vi "Initialise all lasers.vi"() -> (4 "455 laser":refnum<visa-resource-name>, 6 "488 laser":refnum<visa-resource-name>, 8 "561 laser":refnum<visa-resource-name>, 10 "647 laser":refnum<visa-resource-name>, 15 "error out":errorcluster)   [LabVIEW 2017]
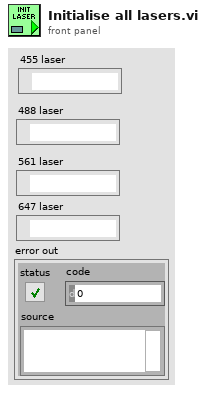
[diagram p1: front panel]
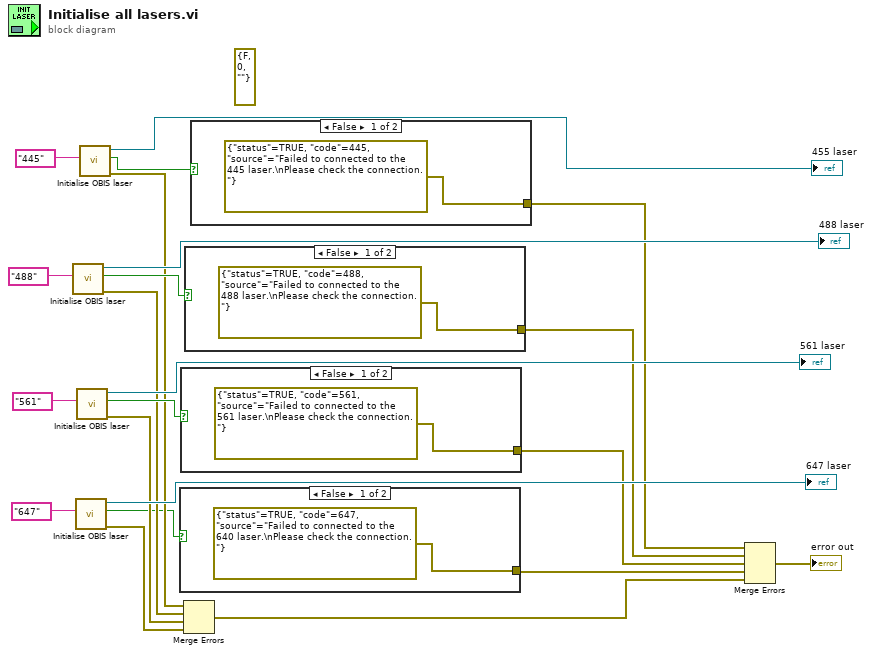
[diagram p0: block diagram]
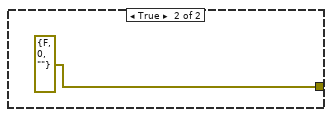
[diagram p2: hidden frame]
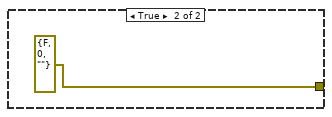
[diagram p3: hidden frame]
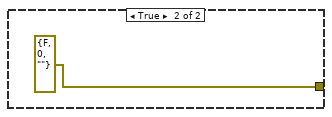
[diagram p4: hidden frame]
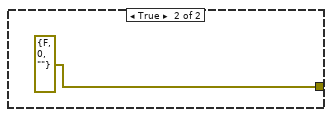
[diagram p5: hidden frame]
diagram:
  (unwired) errorcluster {"status"=FALSE, "code"=0, "source"=""} ("error out")
  n1 = call "Initialise OBIS laser.vi"("Laser to initialise"="488") -> ("error out"=w3:errorcluster, "Connected successfully?"=w13:bool, "VISA resource name out"=→"488 laser":refnum<visa-resource-name>)  [unwired: 8 in]
  n2 = call "Initialise OBIS laser.vi"("Laser to initialise"="647") -> ("error out"=w5:errorcluster, "Connected successfully?"=w1:bool, "VISA resource name out"=→"647 laser":refnum<visa-resource-name>)  [unwired: 8 in]
  n3 = call "Initialise OBIS laser.vi"("Laser to initialise"="561") -> ("error out"=w4:errorcluster, "Connected successfully?"=w12:bool, "VISA resource name out"=→"561 laser":refnum<visa-resource-name>)  [unwired: 8 in]
  n4 = call "Initialise OBIS laser.vi"("Laser to initialise"="445") -> ("error out"=w6:errorcluster, "Connected successfully?"=w15:bool, "VISA resource name out"=→"455 laser":refnum<visa-resource-name>)  [unwired: 8 in]
  n5 = case shown="False" w1 {
    tunnel: [errorcluster {"status"=TRUE, "code"=647, "source"="Failed to connected to the 640 laser.\nPlease check the connection."} ("error out") errorcluster {"status"=FALSE, "code"=0, "source"=""} ("error out")] -> w7
    frame False {
    }
    frame True {
    }
  }
  n6 = case shown="False" w12 {
    tunnel: [errorcluster {"status"=TRUE, "code"=561, "source"="Failed to connected to the 561 laser.\nPlease check the connection."} ("error out") errorcluster {"status"=FALSE, "code"=0, "source"=""} ("error out")] -> w8
    frame False {
    }
    frame True {
    }
  }
  n7 = Merge Errors(w6, w3, w4, w5) -> (w2:errorcluster)
  n8 = case shown="False" w13 {
    tunnel: [errorcluster {"status"=TRUE, "code"=488, "source"="Failed to connected to the 488 laser.\nPlease check the connection."} ("error out") errorcluster {"status"=FALSE, "code"=0, "source"=""} ("error out")] -> w9
    frame False {
    }
    frame True {
    }
  }
  n9 = case shown="False" w15 {
    tunnel: [errorcluster {"status"=TRUE, "code"=445, "source"="Failed to connected to the 445 laser.\nPlease check the connection."} ("error out") errorcluster {"status"=FALSE, "code"=0, "source"=""} ("error out")] -> w10
    frame False {
    }
    frame True {
    }
  }
  n10 = Merge Errors(w10, w9, w8, w7, w2) -> (→"error out":errorcluster)
